vi "Alpha Ver 1.0.vi"() -> ()   [LabVIEW 2015]
uses:
  <instrlib>/Keithley 622x LV 2009/Configure/Source/Typedefs/KE622x -- Current Range.ctl
  <instrlib>/Keithley 622x LV 2009/Configure/Source/Typedefs/KE622x -- Current Ranges.ctl
  <instrlib>/Keithley 622x LV 2009/Typedefs/KE622x -- On Off Control.ctl
  <instrlib>/Keithley 622x LV 2009/Utility/Typedefs/KE622x -- Instrument Type.ctl
  <instrlib>/Keithley 622x LV 2009/Configure/Source/Typedefs/KE622x -- Voltage Limit.ctl
  <instrlib>/Keithley 2000/Public/Configure/Configure DC Volts.vi
  <userlib>/LV-Link3/PolySubVIs/DtCreateAinChan.vi
  <userlib>/LV-Link3/PolySubVIs/DtOLReadSingle.vi
  <instrlib>/Keithley 2000/Keithley 2000.lvlib
  <instrlib>/Keithley 622x LV 2009/Keithley 622x.lvlib
panel:
  out "code":i32
  out "source":string
  out "DAQ A3":dbl format="%#_13g"
  out "DAQ A2":dbl format="%#_13g"
  out "DAQ A1":dbl format="%#_13g"
  out "DAQ cluster":T1
  out "Real stop cur":dbl format="%#_13g"
  out "Real start cur":dbl format="%#_13g"
  in  "Stop cur prefix":u16(ring)
  in  "Start cur prefix":u16(ring)
  out "MULTIPLE GRAPHS":cluster{dbl[], dbl[]}[](graph)
  in  "X-Axis":T2(ring)
  in  "Range":u8(ring)=20 items=["100nV", "200nV", "500nV", "1µV", "2µV", "5µV", "10µV", "20µV", "50µV", "100µV", "200µV", "500µV", "1mV", "2mV", "5mV", "10mV", "20mV", "50mV", "100mV", "200mV", "500mV", "1V"]
  in  "Display Type copy":u16(ring)=3 items=["X %", "Y %", "X Calibrated", "Y Calibrated", "Mag %", "Mag Calibrated", "Phase Degrees", "Ratio", "ADC 1", "ADC 2", "ADC 3", "ADC 4 ", "Noise %", "Noise Calibrated", "Ref Frequency", "", ""]
  out "Units copy":string
  out "Display copy":dbl format="%.3f"
  out "Overload":bool
  out "Display":dbl format="%.3f"
  out "Units":string
  in  "Display Type":u16(ring)=2 items=["X %", "Y %", "X Calibrated", "Y Calibrated", "Mag %", "Mag Calibrated", "Phase Degrees", "Ratio", "ADC 1", "ADC 2", "ADC 3", "ADC 4 ", "Noise %", "Noise Calibrated", "Ref Frequency", "", ""]
  in  "Time Constant":u16(ring) items=["MIN", "1ms", "3ms", "10ms", "30ms", "100ms", "300ms", "1s", "3s", "10s", "30s", "100s", "300s"]
  in  "Slope":u8(ring) items=["6db/octave", "12dB/octave"]
  in  "Dynamic Reserve":u16(ring) items=["High Stability", "Normal", "High Reserve"]
  in  "Auto Sensitivity":bool
  in  "Auto Measure":bool
  out "6221_error_out":errorcluster
  out "2000_error_out":errorcluster
  out "5110_error_out":errorcluster
  out "Input Mode":i32(ring) items=[" Voltage Input (A or A-B) ", "Current Input 10E6 V/A", "Current Input 10E8 V/A"]
  out "5110":refnum<visa-resource-name>
  in  "GPIB Address":i8=11 min=1 max=32 step=1
  out "DAQ A0":dbl format="%#_13g"
  out "2000":dbl format="%#_13g"
  in  "Device":string(combo)
  in  "Number \nof points":i32
  in  "Folder\nprename":string
  out "TIME GRAPH":cluster{dbl[], dbl[]}[](graph)
  out "T0":u32
  out "LIMIT":bool
  out "LIMIT":bool
  out "Error Code":string
  in  "Comments":string
  out "file":refnum<file>
  out "2000":refnum<visa-resource-name>
  out "6221":refnum<visa-resource-name>
  out "Step  (A)":dbl=5e-05 format="%#_3p"
  in  "Stop\ncurrent (A)":dbl=0.002 format="%#_6p"
  in  "Start \ncurrent (A)":dbl=0.001 format="%#_6p"
  in  "Check For SCPI Errors? (T)":bool=TRUE
  out "Interlock Tripped?":bool
  out "Compliance?":bool
  in  "Turn Off Output \nIf Compliance?":bool=TRUE
  in  "Turning ON/OFF\ncurrent output":T3=enum."On"
  in  "Range Selection":T4={"Auto Range?"=TRUE, "Man / Selected\nRange"=enum."2nA"}
  # "FILE CONFIGURATION"
  # "ADMIN PANEL"
  # "KEITHLEY 6221 CONFIGURATION (ADMIN ONLY)"
  # "KEITHLEY DAQ CONFIGURATION (ADMIN ONLY)"
  # "PRINCETON LOCK-IN AMP (ADMIN ONLY)"
  # "I don't know what the hell it is,\njust don't touch it"
  # "SENSITIVITY"
  # "INPUT CONFIGURATION"
  # "READINGS"
  # "START, STOP, STEP, CONFIGURATION"
  # "IF ON"
  # "Output Channels Time - Constant \nSlope & Dynamic Reserve"
  # "Compliance = Limiting output voltage\nThis switch determines if we want to switch \noff the current output if wee exceed compliance"
  # "LOCK-IN READINGS"
  # "RIGHT DISPLAY"
  # "LEFT DISPLAY"
  # "There is a safe switch at \nthe back of the instrument \nThis indicator shows if it is on"
  # "You have hit a damn jackpot \nby exceeding the limited voltage\nCongrats"
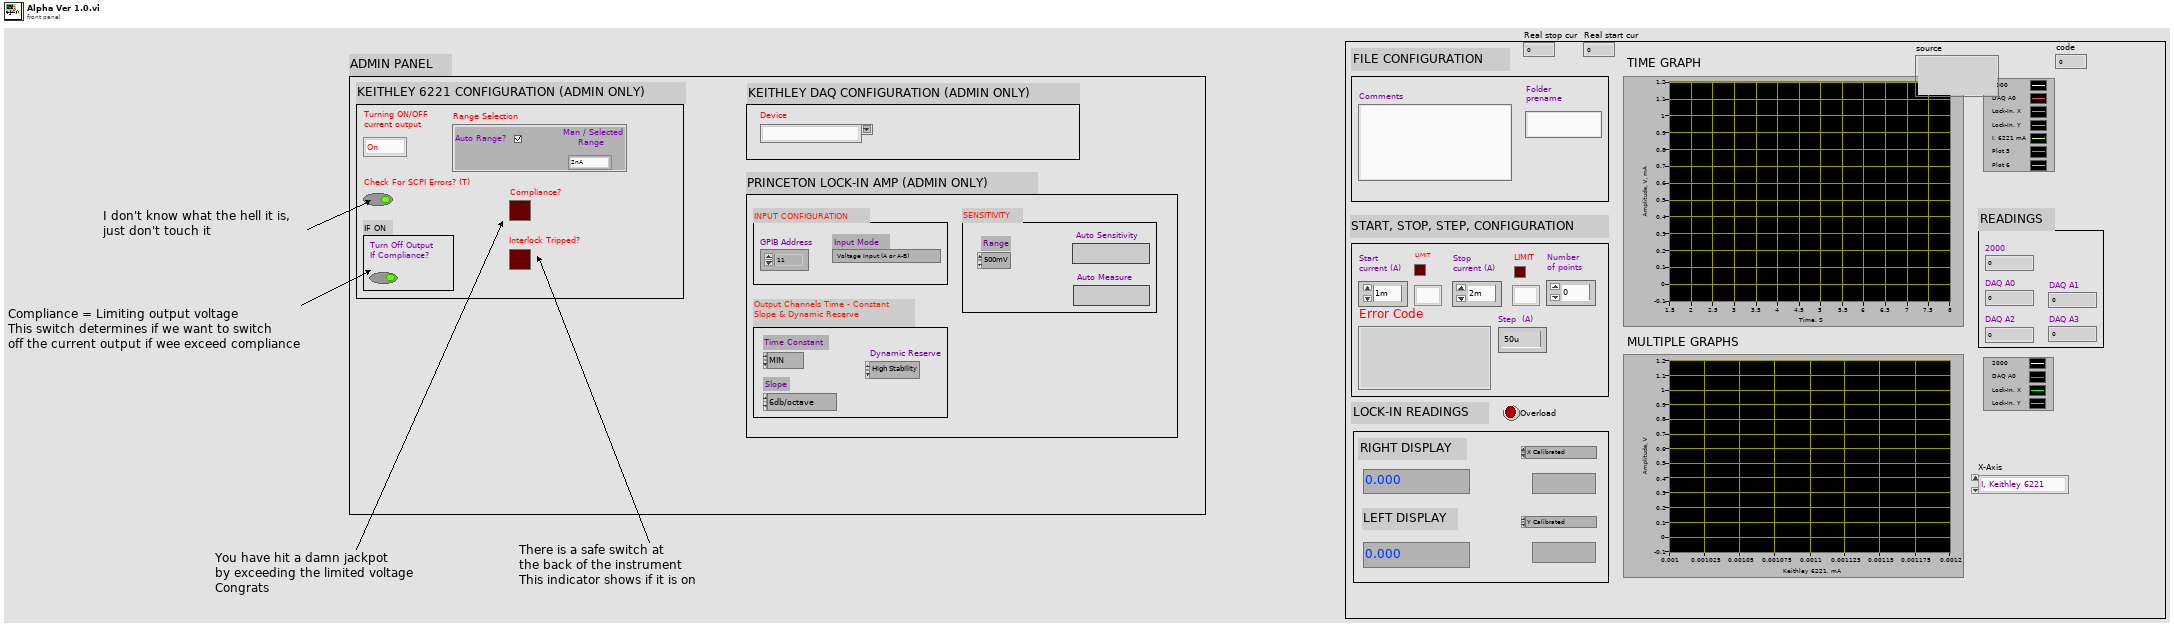
[diagram p1: front panel]
types:
  T1 = cluster{"Task out":i32, "error out":errorcluster, "Task out":i32, "error out":errorcluster, "Task out":i32, "error out":errorcluster, "Task out":i32, "error out":errorcluster}
  T2 = enum16{"I, Keithley 6221", "V, Keithley 2000", "V, Keithley DAQ A0", "V, Keithley DAQ A1", "V, Keithley DAQ A2", "V, Keithley DAQ A3", "V, Lock-In X", "V, Lock-In Y"}
  T3 = typedef "Keithley 622x.lvlib/KE622x -- On Off Control.ctl" = enum16{"Off", "On"}
  T4 = typedef "Keithley 622x.lvlib/KE622x -- Current Range.ctl" = cluster{"Auto Range?":bool, "Man / Selected\nRange":T5}
  T5 = typedef "Keithley 622x.lvlib/KE622x -- Current Ranges.ctl" = enum16{"2nA", "20nA", "200nA", "2uA", "20uA", "200uA", "2mA", "20mA", "100mA"}
  T6 = typedef "Keithley 622x.lvlib/KE622x -- Instrument Type.ctl" = enum16{"KE6220", "KE6221"}
  T7 = typedef "Keithley 622x.lvlib/KE622x -- Voltage Limit.ctl" = dbl
  T8 = cluster{"Data Out":dbl, "Data Out":dbl, "Data Out":dbl, "Data Out":dbl, "Measurement":dbl}
  T9 = cluster{dbl[], dbl[], dbl[], dbl[], dbl[], dbl[], dbl[], dbl[], dbl[]}
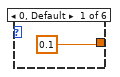
[diagram p2: hidden frame]
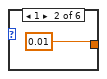
[diagram p3: hidden frame]
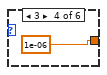
[diagram p4: hidden frame]
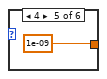
[diagram p5: hidden frame]
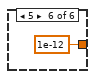
[diagram p6: hidden frame]
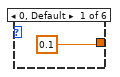
[diagram p7: hidden frame]
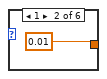
[diagram p8: hidden frame]
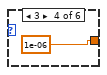
[diagram p9: hidden frame]
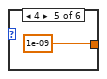
[diagram p10: hidden frame]
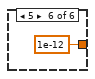
[diagram p11: hidden frame]
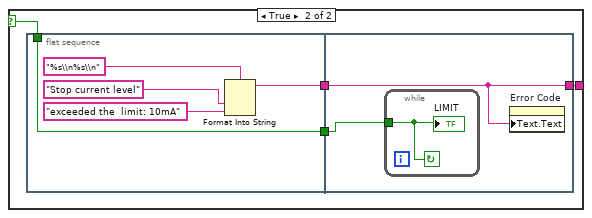
[diagram p12: hidden frame]
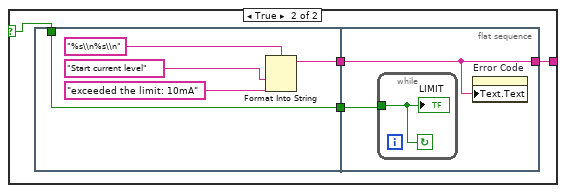
[diagram p13: hidden frame]
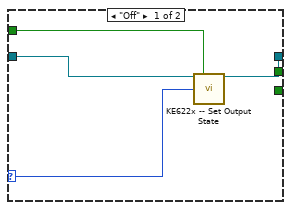
[diagram p14: hidden frame]
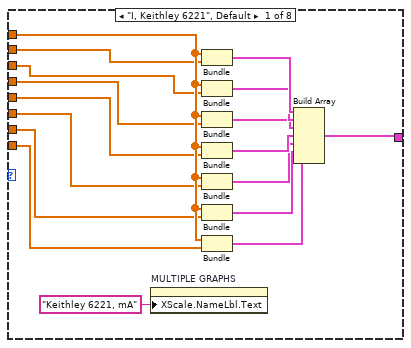
[diagram p15: hidden frame]
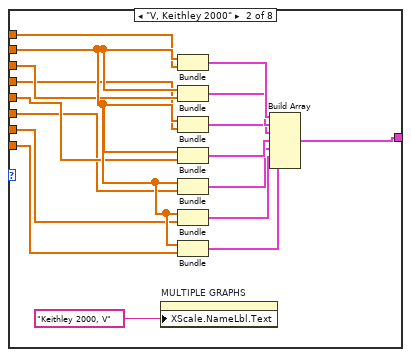
[diagram p16: hidden frame]
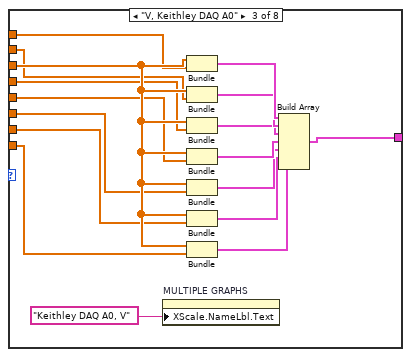
[diagram p17: hidden frame]
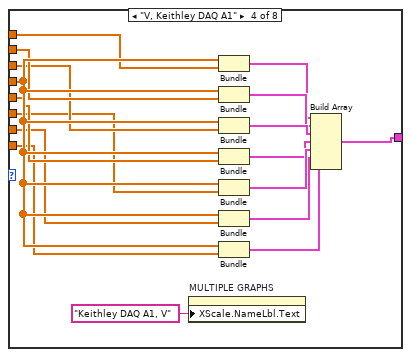
[diagram p18: hidden frame]
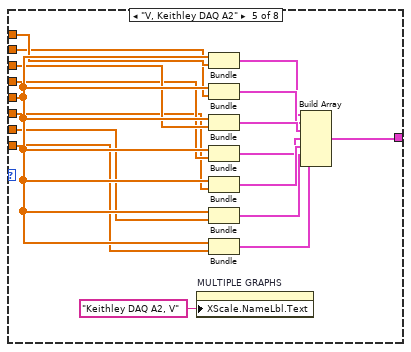
[diagram p19: hidden frame]
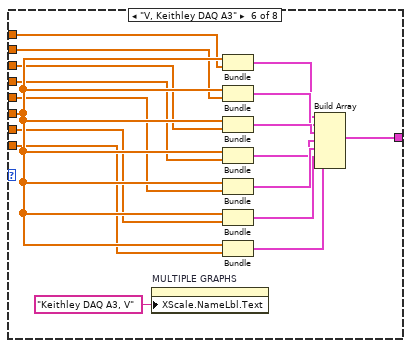
[diagram p20: hidden frame]
diagram:
  n1 = flat-sequence {
    tunnel: [w181] -> w7
    tunnel: [w180] -> w6
    tunnel: [w179] -> w5
    tunnel: [w178] -> w4
    tunnel: [w177] -> w3
    tunnel: [w176] -> w2
    tunnel: [w165] -> w1
    tunnel: w7 -> [w849]
    tunnel: w6 -> [w848]
    tunnel: w5 -> [w847]
    tunnel: w4 -> [w846]
    tunnel: w3 -> [w845]
    tunnel: w2 -> [w844]
    tunnel: w1 -> [w843]
    frame #0 {
      # "File configuration"
      # "Start, Stop, Step"
      # "Time Intit"
      # "Initializing instruments"
      n2 = flat-sequence {
        frame #0 {
          w16 = TRUE  # reset
          w15 = FALSE  # ID query
          # "Initialize Lock-In 5110"
          # "Initialize Keithley 2000"
          # "Initialize Keithley 6221"
          n3 = call <instrlib>:"Initialize.vi"("VISA resource name"=refnum<visa-resource-name> "KEITHLEY_MULTIMETER") -> ("VISA resource name out"=w20:refnum<visa-resource-name>)  [unwired: 17 in, 1 out]
          n4 = call <instrlib>:"Initialize.vi"("VISA resource name"=refnum<visa-resource-name> "KEITHLEY_DC_AC_CURRENT_SOURCE", "Error Queue Option"=enum16{"Clear Error Queue", "Error Query"}."Clear Error Queue", "Instrument Type"=KE622x_--_Instrument_Type."KE6221") -> ("VISA resource name out"=→"6221":refnum<visa-resource-name>, "error out"=→"6221_error_out":errorcluster)  [unwired: 11 in]
          n5 = call "SR51XX Initialize"("VISA session (for class)"=refnum<visa-resource-name> "LOCK_IN_5110_PRINCETON", "Interface"=FALSE, "ID query"=w15, "GPIB Address"="GPIB Address", "reset"=w16) -> ("VISA session"=→"5110":refnum<visa-resource-name>, "error out"=→"5110_error_out":errorcluster)  [unwired: 8 in, 1 out]
          n6 = call-poly <instrlib>:"Configure Measurement.vi"("VISA resource name"=w20) -> ("VISA resource name out"=→"2000":refnum<visa-resource-name>, "error out"=→"2000_error_out":errorcluster)  [unwired: 17 in]
        }
        frame #1 {
          # "Initialize Keithley DAQ \n(getting board name)"
          n7 = call <userlib>:"DtOLGetBoardNames.vi"() -> ("Number of boards"=w25:u32)  [unwired: 9 in, 2 out]
          n8 = Initialize Array("", w25) -> (w27:string[])
          n9 = for {
            N: w25 -> [_]
            shift-right: [w33] -> w30
            shift-left: w27 -> [w34]
            i -> [w32]
            n10 = Add(x=1, y=w32) -> (x+y=w36:i32)
            n11 = call <userlib>:"DtOLGetBoardNames.vi"("Select Board"=w36) -> ("Board Name"=w31:string)  [unwired: 8 in, 2 out]
            n12 = Replace Array Subset(array=w34, new element=w31, index=w32) -> (w33:string[])
          }
          n13 = Index Array(array=w30, index=0) -> (element=w29:string)
          n14 = property on="Device" class="CmbBox"("Strings[]"=w30, "Value"=w29) -> ()  [unwired: 2 in, 2 out]
        }
        frame #2 {
          # "Calculating steps by number\nof points"
          # "Putting in a loop \ninstead of \"STOP\""
          n15 = local read "Real stop cur"() -> (w53:dbl)
          n16 = local read "Real start cur"() -> (w54:dbl)
          n17 = case shown="2" "Start cur prefix" {
            tunnel: [0.1 0.01 0.001 1e-06 1e-09 1e-12] -> w42
            frame 0, Default {
            }
            frame 1 {
            }
            frame 2 {
            }
            frame 3 {
            }
            frame 4 {
            }
            frame 5 {
            }
          }
          n18 = case shown="2" "Stop cur prefix" {
            tunnel: [0.1 0.01 0.001 1e-06 1e-09 1e-12] -> w40
            frame 0, Default {
            }
            frame 1 {
            }
            frame 2 {
            }
            frame 3 {
            }
            frame 4 {
            }
            frame 5 {
            }
          }
          n19 = Subtract(x=w53, y=w54) -> (x-y=w56:dbl)
          n20 = Multiply(x=w42, y="Start \ncurrent (A)") -> (x*y=w38:dbl)
          "Real start cur" <- w38
          n21 = Divide(x=w56, y="Number \nof points") -> (x/y=→"Step  (A)":dbl)
          n22 = Multiply(x=w40, y="Stop\ncurrent (A)") -> (x*y=w37:dbl)
          "Real stop cur" <- w37
          n23 = Greater?(x=w37, y=T7 0.01) -> (0:w48:bool)
          n24 = Greater?(x=w38, y=T7 0.01) -> (0:w47:bool)
          n25 = case shown="False" w48 {
            selector: w48 -> [_ w72]
            tunnel: [w69 w75] -> w50
            frame False {
              n26 = Format Into String(format string="%s\\n", "Start current level is OK" ("false string")) -> (resulting string=w69:string)  [unwired: 2 in, 1 out]
            }
            frame True {
              n27 = flat-sequence {
                tunnel: [w77] -> w74
                tunnel: [w76] -> w73
                tunnel: w72 -> [w76]
                tunnel: [w81] -> w75
                tunnel: w74 -> [w81]
                tunnel: w73 -> [w82]
                frame #0 {
                  n28 = Format Into String(format string="%s\\n%s\\n", "Stop current level" ("String"), "exceeded the  limit: 10mA" ("input 2")) -> (resulting string=w77:string)  [unwired: 2 in, 1 out]
                }
                frame #1 {
                  n29 = while {
                    tunnel: w82 -> [w83]
                    stop <- w83 continue-if-true
                    "LIMIT" <- w83
                  }
                  n30 = property on="Error Code" class="Str"("Text.Text"=w81) -> ()  [unwired: 2 in, 2 out]
                }
              }
            }
          }
          n31 = case shown="False" w47 {
            selector: w47 -> [_ w88]
            tunnel: [w84 w90] -> w49
            frame False {
              n32 = Format Into String(format string="%s\\n", "Start current level is OK" ("false string")) -> (resulting string=w84:string)  [unwired: 2 in, 1 out]
            }
            frame True {
              n33 = flat-sequence {
                tunnel: [w92] -> w89
                tunnel: w88 -> [w91]
                tunnel: [w91] -> w87
                tunnel: [w96] -> w90
                tunnel: w89 -> [w96]
                tunnel: w87 -> [w97]
                frame #0 {
                  n34 = Format Into String(format string="%s\\n%s\\n", "Start current level" ("String"), "exceeded the limit: 10mA" ("input 2")) -> (resulting string=w92:string)  [unwired: 2 in, 1 out]
                }
                frame #1 {
                  n35 = while {
                    tunnel: w97 -> [w98]
                    stop <- w98 continue-if-true
                    "LIMIT" <- w98
                  }
                  n36 = property on="Error Code" class="Str"("Text.Text"=w96) -> ()  [unwired: 2 in, 2 out]
                }
              }
            }
          }
          n37 = Concatenate Strings(w49, w50) -> (→"Error Code":string)
        }
        frame #3 {
          n38 = flat-sequence {
            frame #0 {
              # "Creating folder&file"
              n39 = call "folder_creation.vi"("Name"="Folder\nprename") -> ("String"=w100:string)
              n40 = call "file_creation.vi"("String"=w100) -> ("refnum out"=→"file":refnum<file>)
            }
            frame #1 {
              # "Creating comments"
              n41 = local read "file"() -> (w102:refnum<file>)
              n42 = Format Into String(format string="# %s\\n", initial string=w102, "Comments") -> ()  [unwired: 1 in, 2 out]
            }
            frame #2 {
              # "Writing instr params"
              n43 = local read "5110"() -> (w110:refnum<visa-resource-name>)
              n44 = local read "Real stop cur"() -> (w108:dbl)
              n45 = local read "file"() -> (w105:refnum<file>)
              n46 = local read "Real start cur"() -> (w109:dbl)
              n47 = call "com_inst.vi"("Stop current"=w108, "Start current"=w109, "VISA session (for class)"=w110) -> ("concatenated string"=w106:string)
              n48 = Format Into String(format string="# %s\\n", initial string=w105, w106) -> ()  [unwired: 1 in, 2 out]
            }
            frame #3 {
              # "Adding headlines"
              n49 = local read "file"() -> (w121:refnum<file>)
              n50 = Format Into String(format string="# %-6s  %-12s %-12s %-12s %-12s %-12s  %-12s %-14s %-14s\\n", initial string=w121, "t, ms" ("input 3"), "2000, V" ("input 1"), "DAQ A0" ("input 2"), "DAQ A1" ("input 2"), "DAQ A2" ("input 2"), "DAQ A3" ("input 2"), "5110_X" ("input 3"), "5110_Y " ("input 3"), "6221, mA" ("input 3")) -> ()  [unwired: 1 in, 2 out]
            }
          }
        }
      }
      n51 = Tick Count (ms)() -> (millisecond timer value=→"T0":u32)
    }
    frame #1 {
      # "Configuring Keithley DAQ just before measuments"
      # "Configuring Keithley 6221 just before measuments"
      n52 = flat-sequence {
        tunnel: [w140] -> w122
        tunnel: [w158] -> _
        tunnel: [w160] -> _
        tunnel: w122 -> [w159]
        frame #0 {
          # "Current range \nselection check"
          # "Checking for compliance\nand interlock errors"
          n53 = local read "6221"() -> (w143:refnum<visa-resource-name>)
          n54 = call <instrlib>:"KE622x -- Set Current Range.vi"("Resource In"=w143, "Current Range In"="Range Selection", "Read Back Set Values? (T)"=FALSE) -> ("Resource Out (dupl)"=w148:refnum<visa-resource-name>)  [unwired: 10 in, 2 out]
          n55 = case shown="\"On\"" "Turning ON/OFF\ncurrent output" {
            selector: "Turning ON/OFF\ncurrent output" -> [w152 _]
            tunnel: [_ w156] -> w146
            tunnel: [_ w155] -> w147
            tunnel: "Check For SCPI Errors? (T)" -> [w151 _]
            tunnel: w148 -> [w149 w154]
            tunnel: [w150 w153] -> w140
            frame "Off" {
              n56 = call <instrlib>:"KE622x -- Set Output State.vi"("Resource In"=w149, "Check For SCPI Errors? (T)"=w151, "Output State"=w152) -> ("Resource Out (dupl)"=w150:refnum<visa-resource-name>)  [unwired: 11 in, 1 out]
            }
            frame "On" {
              n57 = call <instrlib>:"KE622x -- Turn Output On And Check For Errors.vi"("Resource In"=w154, "Turn Off Output If Compliance?"="Turn Off Output \nIf Compliance?") -> ("Resource Out (dupl)"=w153:refnum<visa-resource-name>, "Interlock Tripped?"=w156:bool, "Compliance?"=w155:bool)  [unwired: 10 in, 1 out]
            }
          }
          "Interlock Tripped?" <- w146
          "Compliance?" <- w147
        }
        frame #1 {
          # "Setting start current"
          n58 = local read "Real start cur"() -> (w158:dbl)
          n59 = Wait (ms)(milliseconds to wait=u32 100) -> ()  [unwired: 1 out]
          n60 = call <instrlib>:"KE622x -- Set Current Level.vi"("Resource In"=w159, "Current Level (A) In"=w158) -> ("Resource Out (dupl)"=w160:refnum<visa-resource-name>)  [unwired: 12 in, 1 out]
        }
      }
      n61 = flat-sequence {
        frame #0 {
          w134 = 10.0 ("Range Max")
          w133 = -10.0 ("Range Min")
          w135 = 100 items=["SingleEnded"=100, "Differential"=101] ("Channel Type")
          # "Configure the input channel"
          n62 = call-poly <userlib>:"DtOLCreateTask.vi"("Channel Type"=w135, "Range Min"=w133, "Range Max"=w134, "Board Name"="Device", "Channel"="0" ("Channels")) -> ("Task out"=w131:i32, "error out"=w130:errorcluster)  [unwired: 8 in, 1 out]
          n63 = call-poly <userlib>:"DtOLCreateTask.vi"("Channel Type"=w135, "Range Min"=w133, "Range Max"=w134, "Board Name"="Device", "Channel"="1") -> ("Task out"=w129:i32, "error out"=w128:errorcluster)  [unwired: 8 in, 1 out]
          n64 = call-poly <userlib>:"DtOLCreateTask.vi"("Channel Type"=w135, "Range Min"=w133, "Range Max"=w134, "Board Name"="Device", "Channel"="2") -> ("Task out"=w127:i32, "error out"=w126:errorcluster)  [unwired: 8 in, 1 out]
          n65 = call-poly <userlib>:"DtOLCreateTask.vi"("Channel Type"=w135, "Range Min"=w133, "Range Max"=w134, "Board Name"="Device", "Channel"="3") -> ("Task out"=w125:i32, "error out"=w124:errorcluster)  [unwired: 8 in, 1 out]
          n66 = Bundle("Task out"=w131, "error out"=w130, "Task out"=w129, "error out"=w128, "Task out"=w127, "error out"=w126, "Task out"=w125, "error out"=w124) -> (→"DAQ cluster":T1)  [unwired: 1 in]
        }
      }
    }
    frame #2 {
      n67 = local read "5110"() -> (w172:refnum<visa-resource-name>)
      n68 = local read "2000"() -> (w171:refnum<visa-resource-name>)
      n69 = local read "6221"() -> (w170:refnum<visa-resource-name>)
      n70 = local read "5110_error_out"() -> (w169:errorcluster)
      n71 = local read "6221_error_out"() -> (w168:errorcluster)
      n72 = local read "2000_error_out"() -> (w167:errorcluster)
      n73 = local read "DAQ cluster"() -> (w166:T1)
      n74 = while {
        shift-right: [w276] -> _
        shift-left: dbl[] [] -> [w444]
        shift-right: [w277] -> _
        shift-left: i32[] [] -> [w443]
        tunnel: w171 -> [w441]
        tunnel: w170 -> [w440]
        shift-right: [w272] -> _
        shift-left: dbl[] [] -> [w433]
        tunnel: [w432] -> w181
        tunnel: [w431] -> w180
        tunnel: [w429] -> w179
        tunnel: [w426] -> w178
        tunnel: w172 -> [w422]
        tunnel: w169 -> [w421]
        tunnel: w168 -> [w413]
        tunnel: w167 -> [w412]
        tunnel: [w363] -> w177
        tunnel: [w360] -> w176
        shift-right: [w271] -> _
        shift-left: dbl[] [] -> [w359]
        shift-right: [w270] -> _
        shift-left: dbl[] [] -> [w358]
        shift-right: [w278] -> _
        shift-left: dbl[] [] -> [w355]
        tunnel: w166 -> [w312]
        tunnel: [w308] -> w165
        shift-right: [w275] -> _
        shift-left: dbl[] [] -> [w307]
        shift-right: [w274] -> _
        shift-left: dbl[] [] -> [w306]
        shift-right: [w273] -> _
        shift-left: dbl[] [] -> [w305]
        i -> [w414]
        stop <- w434 stop-if-true
        # "V, DAQ A3"
        # "V, DAQ A2"
        # "V, DAQ A1"
        # "Y-V, 5110"
        # "X-V, 5110"
        # "I, 6221"
        # "Config delay"
        # "Control subVI 5110"
        # "Read config 5110"
        # "Measurement config 5110"
        # "Time config 5110"
        # "Configuring Right Display 5110"
        # "Configuring Left Display 5110"
        # "Setting 6221 current"
        # "Delay before measuremens"
        # "Getting the data from DAQ and 2000"
        # "Changing input current"
        # "Time"
        # "V, DAQ A0"
        # "V, 2000"
        n75 = local read "T0"() -> (w442:u32)
        n76 = Quotient & Remainder(x=w414, y=10) -> (floor(x/y)=w419:i32)  [unwired: 1 out]
        n77 = Equal?(x=0, y=w414) -> (x = y?=w416:bool)
        n78 = Subtract(x=w403, y=w442) -> (x-y=w323:u32)
        n79 = Equal?(x=1, y=w419) -> (x = y?=w415:bool)
        n80 = flat-sequence {
          tunnel: w441 -> [w591]
          tunnel: [w591] -> w354
          tunnel: w440 -> [w590]
          tunnel: [w590] -> w352
          tunnel: w422 -> [w588]
          tunnel: [w588] -> w350
          tunnel: [w587] -> w348
          tunnel: w421 -> [w587]
          tunnel: w416 -> [w586]
          tunnel: [w586] -> w346
          tunnel: w415 -> [w585]
          tunnel: [w585] -> w344
          tunnel: w413 -> [w584]
          tunnel: [w584] -> w342
          tunnel: w412 -> [w583]
          tunnel: [w583] -> w340
          tunnel: [w582] -> w403
          tunnel: [w581] -> w313
          tunnel: w312 -> [w581]
          tunnel: w354 -> [w606]
          tunnel: [w606] -> w353
          tunnel: w352 -> [w605]
          tunnel: [w605] -> w351
          tunnel: w350 -> [w604]
          tunnel: [w604] -> w349
          tunnel: w348 -> [w603]
          tunnel: [w603] -> w347
          tunnel: w346 -> [w602]
          tunnel: [w602] -> w345
          tunnel: w344 -> [w601]
          tunnel: [w601] -> w343
          tunnel: w342 -> [w600]
          tunnel: [w600] -> w341
          tunnel: w340 -> [w599]
          tunnel: [w599] -> w339
          tunnel: [w592] -> w314
          tunnel: w313 -> [w592]
          tunnel: w353 -> [w619]
          tunnel: [w619] -> w402
          tunnel: w351 -> [w618]
          tunnel: [w618] -> w401
          tunnel: w349 -> [w617]
          tunnel: w347 -> [w614]
          tunnel: [w613] -> w400
          tunnel: [w612] -> w399
          tunnel: w345 -> [w611]
          tunnel: [w611] -> w398
          tunnel: w343 -> [w610]
          tunnel: w341 -> [w609]
          tunnel: [w609] -> w397
          tunnel: w339 -> [w608]
          tunnel: [w608] -> w396
          tunnel: [w607] -> w315
          tunnel: w314 -> [w607]
          tunnel: w402 -> [w644]
          tunnel: [w644] -> w395
          tunnel: w401 -> [w643]
          tunnel: [w643] -> w394
          tunnel: w400 -> [w640]
          tunnel: [w639] -> w393
          tunnel: w399 -> [w638]
          tunnel: [w637] -> w392
          tunnel: w398 -> [w635]
          tunnel: [w635] -> w391
          tunnel: w397 -> [w642]
          tunnel: [w642] -> w390
          tunnel: w396 -> [w641]
          tunnel: [w641] -> w389
          tunnel: ["Auto Measure"] -> w388
          tunnel: ["Auto Sensitivity"] -> w387
          tunnel: [w630] -> w386
          tunnel: [w627] -> w316
          tunnel: w315 -> [w627]
          tunnel: w395 -> [w663]
          tunnel: [w663] -> w338
          tunnel: w394 -> [w662]
          tunnel: [w662] -> w337
          tunnel: w393 -> [w655]
          tunnel: w392 -> [w653]
          tunnel: [w652] -> w336
          tunnel: w391 -> [w659]
          tunnel: [w659] -> w335
          tunnel: w390 -> [w661]
          tunnel: [w661] -> w334
          tunnel: w389 -> [w660]
          tunnel: [w660] -> w333
          tunnel: w388 -> [w657]
          tunnel: [w657] -> w332
          tunnel: w387 -> [w658]
          tunnel: [w658] -> w331
          tunnel: w386 -> [w648]
          tunnel: [w648] -> w330
          tunnel: [w654] -> w329
          tunnel: ["Time Constant"] -> w328
          tunnel: ["Slope"] -> w327
          tunnel: [w645] -> w317
          tunnel: w316 -> [w645]
          tunnel: [w687] -> w385
          tunnel: [w686] -> w384
          tunnel: [w672] -> w383
          tunnel: [w685] -> w382
          tunnel: [w684] -> w381
          tunnel: [w683] -> w380
          tunnel: [w682] -> w379
          tunnel: [w681] -> w378
          tunnel: [w674] -> w377
          tunnel: [w677] -> w376
          tunnel: [w675] -> w375
          tunnel: [w680] -> w374
          tunnel: [w665] -> w293
          tunnel: w327 -> [w680]
          tunnel: w328 -> [w675]
          tunnel: w329 -> [w678]
          tunnel: w330 -> [w674]
          tunnel: w331 -> [w681]
          tunnel: w332 -> [w682]
          tunnel: w333 -> [w683]
          tunnel: w334 -> [w684]
          tunnel: w335 -> [w685]
          tunnel: w336 -> [w673]
          tunnel: w337 -> [w686]
          tunnel: w338 -> [w687]
          tunnel: [w664] -> w318
          tunnel: w317 -> [w664]
          tunnel: w385 -> [w711]
          tunnel: [w711] -> w373
          tunnel: w384 -> [w710]
          tunnel: [w710] -> w372
          tunnel: w383 -> [w697]
          tunnel: w382 -> [w709]
          tunnel: [w709] -> w371
          tunnel: w381 -> [w708]
          tunnel: [w708] -> w370
          tunnel: w380 -> [w707]
          tunnel: [w707] -> w369
          tunnel: w379 -> [w706]
          tunnel: [w706] -> w368
          tunnel: w378 -> [w705]
          tunnel: [w705] -> w367
          tunnel: w377 -> [w698]
          tunnel: w376 -> [w695]
          tunnel: [w694] -> w366
          tunnel: w375 -> [w699]
          tunnel: w374 -> [w700]
          tunnel: [w696] -> w365
          tunnel: [w693] -> w364
          tunnel: [w689] -> w292
          tunnel: [w688] -> w319
          tunnel: w318 -> [w688]
          tunnel: [w715] -> w438
          tunnel: w414 -> [w723]
          tunnel: [w719] -> w434
          tunnel: [w713] -> w436
          tunnel: [w721] -> w435
          tunnel: [w718] -> w411
          tunnel: [w717] -> w410
          tunnel: [w716] -> w409
          tunnel: [w714] -> w408
          tunnel: [w713] -> w294
          tunnel: w364 -> [_]
          tunnel: w365 -> [w716]
          tunnel: w366 -> [w714]
          tunnel: w367 -> [_]
          tunnel: w368 -> [_]
          tunnel: w369 -> [w718]
          tunnel: w370 -> [w717]
          tunnel: w371 -> [_]
          tunnel: w372 -> [w721]
          tunnel: w373 -> [w715]
          tunnel: [w712] -> w320
          tunnel: w319 -> [w712]
          tunnel: w438 -> [w735]
          tunnel: [w735] -> w437
          tunnel: w436 -> [w734]
          tunnel: w435 -> [w733]
          tunnel: [w732] -> w430
          tunnel: [w731] -> w427
          tunnel: w411 -> [w729]
          tunnel: w410 -> [w730]
          tunnel: w409 -> [w727]
          tunnel: w408 -> [w728]
          tunnel: [w729] -> w407
          tunnel: [w728] -> w404
          tunnel: [w727] -> w361
          tunnel: [w726] -> w321
          tunnel: w320 -> [w726]
          tunnel: w437 -> [w743]
          tunnel: [w743] -> w439
          tunnel: w430 -> [w741]
          tunnel: [w741] -> w428
          tunnel: w427 -> [w740]
          tunnel: [w740] -> w425
          tunnel: w407 -> [w739]
          tunnel: [w739] -> w406
          tunnel: [w738] -> w405
          tunnel: w404 -> [w738]
          tunnel: [w737] -> w362
          tunnel: w361 -> [w737]
          tunnel: [w736] -> w322
          tunnel: w321 -> [w736]
          tunnel: w439 -> [w778]
          tunnel: w428 -> [w774]
          tunnel: w425 -> [w773]
          tunnel: w406 -> [w770]
          tunnel: w405 -> [w769]
          tunnel: w362 -> [w768]
          tunnel: w322 -> [w767]
          tunnel: [w771] -> w235
          tunnel: [w772] -> w234
          tunnel: [w776] -> w233
          tunnel: [w775] -> w232
          tunnel: [w774] -> w231
          tunnel: [w773] -> w230
          tunnel: [w772] -> w229
          tunnel: [w771] -> w228
          tunnel: [w769] -> w227
          tunnel: [w768] -> w226
          tunnel: [w746] -> w225
          tunnel: [w745] -> w224
          tunnel: [w744] -> w223
          tunnel: [w747] -> w222
          tunnel: [w746] -> w221
          tunnel: [w745] -> w220
          tunnel: [w744] -> w219
          tunnel: w235 -> [w795]
          tunnel: w234 -> [w794]
          tunnel: w233 -> [w793]
          tunnel: w232 -> [w792]
          tunnel: w231 -> [w791]
          tunnel: w230 -> [w790]
          tunnel: w229 -> [w789]
          tunnel: w228 -> [w788]
          tunnel: w227 -> [w787]
          tunnel: w226 -> [w786]
          tunnel: w225 -> [w785]
          tunnel: w224 -> [w784]
          tunnel: w223 -> [w783]
          tunnel: w222 -> [w782]
          tunnel: w221 -> [w781]
          tunnel: w220 -> [w780]
          tunnel: w219 -> [w779]
          tunnel: [w795] -> w218
          tunnel: [w794] -> w217
          tunnel: [w793] -> w216
          tunnel: [w792] -> w215
          tunnel: [w791] -> w214
          tunnel: [w790] -> w213
          tunnel: [w789] -> w212
          tunnel: [w788] -> w211
          tunnel: [w787] -> w210
          tunnel: [w786] -> w209
          tunnel: [w785] -> w208
          tunnel: [w784] -> w207
          tunnel: [w783] -> w206
          tunnel: [w782] -> w205
          tunnel: [w781] -> w204
          tunnel: [w780] -> w203
          tunnel: [w779] -> w202
          tunnel: w218 -> [w812]
          tunnel: w217 -> [w811]
          tunnel: w216 -> [w810]
          tunnel: w215 -> [w809]
          tunnel: w214 -> [w808]
          tunnel: w213 -> [w807]
          tunnel: w212 -> [w806]
          tunnel: w211 -> [w805]
          tunnel: w210 -> [w804]
          tunnel: w209 -> [w803]
          tunnel: w208 -> [w802]
          tunnel: w207 -> [w801]
          tunnel: w206 -> [w800]
          tunnel: w205 -> [w799]
          tunnel: w204 -> [w798]
          tunnel: w203 -> [w797]
          tunnel: w202 -> [w796]
          tunnel: [w812] -> w201
          tunnel: [w811] -> w200
          tunnel: [w810] -> w199
          tunnel: [w809] -> w198
          tunnel: [w808] -> w197
          tunnel: [w807] -> w196
          tunnel: [w806] -> w195
          tunnel: [w805] -> w194
          tunnel: [w804] -> w193
          tunnel: [w803] -> w192
          tunnel: [w802] -> w191
          tunnel: [w801] -> w190
          tunnel: [w800] -> w189
          tunnel: [w799] -> w188
          tunnel: [w798] -> w187
          tunnel: [w797] -> w186
          tunnel: [w796] -> w185
          tunnel: [w813] -> w301
          tunnel: [w814] -> w302
          tunnel: [w815] -> w303
          tunnel: [w816] -> w308
          tunnel: [w817] -> w309
          tunnel: [w818] -> w310
          tunnel: [w819] -> w311
          tunnel: [w820] -> w360
          tunnel: [w821] -> w363
          tunnel: [w822] -> w423
          tunnel: [w823] -> w424
          tunnel: [w824] -> w426
          tunnel: [w825] -> w429
          tunnel: [w826] -> w431
          tunnel: [w827] -> w432
          tunnel: [w828] -> w304
          tunnel: [w829] -> w300
          tunnel: w201 -> [w829]
          tunnel: w200 -> [w828]
          tunnel: w199 -> [w827]
          tunnel: w198 -> [w826]
          tunnel: w197 -> [w825]
          tunnel: w196 -> [w824]
          tunnel: w195 -> [w823]
          tunnel: w194 -> [w822]
          tunnel: w193 -> [w821]
          tunnel: w192 -> [w820]
          tunnel: w191 -> [w819]
          tunnel: w190 -> [w818]
          tunnel: w189 -> [w817]
          tunnel: w188 -> [w816]
          tunnel: w187 -> [w815]
          tunnel: w186 -> [w814]
          tunnel: w185 -> [w813]
          frame #0 {
            n81 = Wait Until Next ms Multiple(millisecond multiple=u32 500) -> (millisecond timer value=w582:u32)
          }
          frame #1 {
            n82 = control-ref of="Range"() -> (w598:refnum<vi>)
            n83 = control-ref of="Auto Sensitivity"() -> (w597:refnum<vi>)
            n84 = control-ref of="Auto Measure"() -> (w596:refnum<vi>)
            n85 = control-ref of="Time Constant"() -> (w593:refnum<vi>)
            n86 = control-ref of="Slope"() -> (w594:refnum<vi>)
            n87 = control-ref of="Dynamic Reserve"() -> (w595:refnum<vi>)
            n88 = call "cont_ver_1.0.vi"("Dynamic Reserve"=w595, "Slope"=w594, "Time Constant"=w593, "Auto Measure"=w596, "Auto Sensitivity"=w597, "Range"=w598) -> ()
          }
          frame #2 {
            n89 = case shown="False" w610 {
              tunnel: w617 -> [w621 w626]
              tunnel: [w620 w624] -> w616
              tunnel: [w621 w623] -> w615
              tunnel: w614 -> [w620 w622]
              frame False {
              }
              frame True {
                n90 = call "SR51XX Read Preamp Input Mode"("VISA session (for class)"=w626, "error in (no error)"=w622) -> ("VISA session"=w623:refnum<visa-resource-name>, "Input Mode"=w625:i32, "error out"=w624:errorcluster)  [unwired: 15 in]
                n91 = local write "Input Mode"(w625) -> ()
              }
            }
            n92 = call "SR51XX Configure Signal Channel Input"("VISA session (for class)"=w615, "error in (no error)"=w616, "Update"=w611) -> ("VISA session"=w613:refnum<visa-resource-name>, "error out"=w612:errorcluster)  [unwired: 15 in]
          }
          frame #3 {
            n93 = local read "Input Mode"() -> (w636:i32)
            n94 = call "SR51XX Configure Sensitivity"("VISA session (for class)"=w640, "Input Mode"=w636, "Range"="Range", "error in (no error)"=w638, "Auto Sensitivity"="Auto Sensitivity", "Auto Measure"="Auto Measure", "Update"=w635) -> ("Range Annotations Out[]"=w628:string[], "VISA session"=w639:refnum<visa-resource-name>, "Auto Sensitivity out"=w632:bool, "Auto Measure out"=w631:bool, "Range Out"=w630:u8, "error out"=w637:errorcluster)  [unwired: 7 in]
            n95 = property on="Range" class="Ring (strict)"("Strings []"=w628) -> ()  [unwired: 2 in, 2 out]
            n96 = local write "Auto Sensitivity"(w632) -> ()
            n97 = local write "Auto Measure"(w631) -> ()
            n98 = local write "Range"(w630) -> ()
          }
          frame #4 {
            n99 = Or(x=w658, y=w657) -> (x .or. y?=w656:bool)
            n100 = call "SR51XX Configure Output Channels - Slope, TC and Dyn Reserve"("VISA session (for class)"=w655, "Time Constant"="Time Constant", "Slope"="Slope", "Check TC"=w656, "Dynamic Reserve"="Dynamic Reserve", "error in (no error)"=w653, "Range"=w648, "Update"=w659) -> ("VISA session"=w654:refnum<visa-resource-name>, "Slope Out"=w649:u8, "Time Constant Out"=w650:u16, "error out"=w652:errorcluster)  [unwired: 8 in]
            n101 = local write "Slope"(w649) -> ()
            n102 = local write "Time Constant"(w650) -> ()
          }
          frame #5 {
            n103 = local read "Input Mode"() -> (w679:i32)
            n104 = call "SR5110 Read Output"("VISA session (for class)"=w678, "Input Mode"=w679, "Time Constant"=w675, "Display Type"="Display Type", "Range"=w674, "error in (no error)"=w673, "Slope"=w680) -> ("Units"=w667:string, "Display Precision"=w671:i32, "Display"=w666:dbl, "VISA session"=w677:refnum<visa-resource-name>, "Available Display Types Out"=w670:string[], "Overload"=→"Overload":bool, "error out"=w672:errorcluster)  [unwired: 4 in, 2 out]
            "Units" <- w667
            "Display" <- w666
            n105 = property on="Display Type" class="Ring (strict)"("Strings []"=w670) -> ()  [unwired: 2 in, 2 out]
            n106 = property on="Display" class="DigNum (strict)"("Precision"=w671) -> ()  [unwired: 2 in, 2 out]
            n107 = call "pref_to_num.vi"("string"=w667) -> ("Numeric"=w668:dbl)
            n108 = Multiply(x=w668, y=w666) -> (x*y=w665:dbl)
          }
          frame #6 {
            n109 = local read "Input Mode"() -> (w704:i32)
            n110 = call "SR5110 Read Output"("VISA session (for class)"=w695, "Input Mode"=w704, "Time Constant"=w699, "Display Type"="Display Type copy", "Range"=w698, "error in (no error)"=w697, "Slope"=w700) -> ("Units"=w692:string, "Display Precision"=w701:i32, "Display"=w691:dbl, "VISA session"=w694:refnum<visa-resource-name>, "Reference Unlock"=w693:bool, "Available Display Types Out"=w702:string[], "error out"=w696:errorcluster)  [unwired: 4 in, 2 out]
            "Display copy" <- w691
            "Units copy" <- w692
            n111 = property on="Display Type copy" class="Ring (strict)"("Strings []"=w702) -> ()  [unwired: 2 in, 2 out]
            n112 = property on="Display copy" class="DigNum (strict)"("Precision"=w701) -> ()  [unwired: 2 in, 2 out]
            n113 = call "pref_to_num.vi"("string"=w692) -> ("Numeric"=w690:dbl)
            n114 = Multiply(x=w690, y=w691) -> (x*y=w689:dbl)
          }
          frame #7 {
            n115 = local read "Step  (A)"() -> (w724:dbl)
            n116 = local read "Real start cur"() -> (w725:dbl)
            n117 = Multiply(x=w724, y=w723) -> (x*y=w722:dbl)
            n118 = Add(x=w725, y=w722) -> (x+y=w713:dbl)
            n119 = local read "Real stop cur"() -> (w720:dbl)
            n120 = Greater Or Equal?(x=w713, y=w720) -> (x >= y?=w719:bool)
          }
          frame #8 {
            n121 = call <instrlib>:"KE622x -- Set Current Level.vi"("Resource In"=w733, "Current Level (A) In"=w734, "error in (no error)"=w730) -> ("Resource Out (dupl)"=w731:refnum<visa-resource-name>, "error out"=w732:errorcluster)  [unwired: 11 in]
          }
          frame #9 {
            n122 = Wait Until Next ms Multiple(millisecond multiple=u32 50) -> ()  [unwired: 1 out]
          }
          frame #10 {
            n123 = Unbundle(w767) -> ("Task out"=w766:i32, "error out"=w765:errorcluster, "Task out"=w763:i32, "error out"=w762:errorcluster, "Task out"=w760:i32, "error out"=w759:errorcluster, "Task out"=w758:i32, "error out"=w757:errorcluster)
            n124 = call <instrlib>:"Data Read Single.vi"("VISA resource name"=w778, "error in (no error)"=w770) -> ("VISA resource name out"=w775:refnum<visa-resource-name>, "Measurement"=w771:dbl, "error out"=w776:errorcluster)  [unwired: 13 in, 2 out]
            n125 = call-poly <userlib>:"DtOLRead.vi"("error in (no error)"=w765, "Timeout"=1.0, "Task in"=w766) -> ("error out"=w754:errorcluster, "Data Out"=w772:dbl, "Task out"=w755:i32)  [unwired: 6 in]
            n126 = call-poly <userlib>:"DtOLRead.vi"("error in (no error)"=w757, "Timeout"=1.0, "Task in"=w758) -> ("error out"=w748:errorcluster, "Data Out"=w744:dbl, "Task out"=w749:i32)  [unwired: 6 in]
            n127 = call-poly <userlib>:"DtOLRead.vi"("error in (no error)"=w762, "Timeout"=1.0, "Task in"=w763) -> ("error out"=w752:errorcluster, "Data Out"=w746:dbl, "Task out"=w753:i32)  [unwired: 6 in]
            n128 = call-poly <userlib>:"DtOLRead.vi"("error in (no error)"=w759, "Timeout"=1.0, "Task in"=w760) -> ("error out"=w750:errorcluster, "Data Out"=w745:dbl, "Task out"=w751:i32)  [unwired: 6 in]
            n129 = Bundle("Task out"=w755, "error out"=w754, "Task out"=w753, "error out"=w752, "Task out"=w751, "error out"=w750, "Task out"=w749, "error out"=w748) -> (w747:T1)  [unwired: 1 in]
          }
          frame #11 {
          }
          frame #12 {
          }
          frame #13 {
          }
        }
        n130 = Divide(x=w323, y=u32 1000) -> (x/y=w324:dbl)
        n131 = Build Array (concatenate)(w443, w324) -> (w286:dbl[])
        n132 = local read "file"() -> (w326:refnum<file>)
        n133 = Bundle(w294, w293, w292) -> (w291:cluster{dbl, dbl, dbl})  [unwired: 1 in]
        n134 = Unbundle(w291) -> (w290:dbl, w289:dbl, w288:dbl)
        n135 = Build Array (concatenate)(w355, w290) -> (w287:dbl[])
        n136 = Build Array (concatenate)(w359, w289) -> (w280:dbl[])
        n137 = Build Array (concatenate)(w358, w288) -> (w279:dbl[])
        n138 = Bundle("Data Out"=w304, "Data Out"=w303, "Data Out"=w302, "Data Out"=w301, "Measurement"=w300) -> (w241:T8)  [unwired: 1 in]
        n139 = Unbundle(w241) -> ("Data Out"=w298:dbl, "Data Out"=w297:dbl, "Data Out"=w296:dbl, "Data Out"=w295:dbl, "Measurement"=w299:dbl)
        n140 = Unbundle(w241) -> ("Data Out"=w239:dbl, "Data Out"=w238:dbl, "Data Out"=w237:dbl, "Data Out"=w236:dbl, "Measurement"=w240:dbl)
        n141 = Build Array (concatenate)(w444, w299) -> (w285:dbl[])
        n142 = Build Array (concatenate)(w307, w298) -> (w284:dbl[])
        n143 = Build Array (concatenate)(w306, w297) -> (w283:dbl[])
        n144 = Build Array (concatenate)(w305, w296) -> (w282:dbl[])
        n145 = Build Array (concatenate)(w433, w295) -> (w281:dbl[])
        n146 = Format Into String(format string="%08d  %8.2e %12g %14.5e %12.4e %12.4e\\n", initial string=w326, w323, w240, w239, w238, w237, w236) -> ()  [unwired: 1 in, 2 out]
        n147 = Bundle(w287, w286, w285, w284, w283, w282, w281, w280, w279) -> (w251:T9)  [unwired: 1 in]
        n148 = Unbundle(w251) -> (w261:dbl[], w269:dbl[], w268:dbl[], w267:dbl[], w266:dbl[], w265:dbl[], w264:dbl[], w263:dbl[], w262:dbl[])
        n149 = Bundle(w269, w268) -> (w260:cluster{dbl[], dbl[]})  [unwired: 1 in]
        n150 = Bundle(w269, w267) -> (w259:cluster{dbl[], dbl[]})  [unwired: 1 in]
        n151 = Bundle(w269, w266) -> (w258:cluster{dbl[], dbl[]})  [unwired: 1 in]
        n152 = Bundle(w269, w265) -> (w257:cluster{dbl[], dbl[]})  [unwired: 1 in]
        n153 = Bundle(w269, w264) -> (w256:cluster{dbl[], dbl[]})  [unwired: 1 in]
        n154 = Bundle(w269, w263) -> (w255:cluster{dbl[], dbl[]})  [unwired: 1 in]
        n155 = Bundle(w269, w262) -> (w254:cluster{dbl[], dbl[]})  [unwired: 1 in]
        n156 = Bundle(w269, w261) -> (w253:cluster{dbl[], dbl[]})  [unwired: 1 in]
        n157 = Build Array(w260, w259, w258, w257, w256, w255, w254, w253) -> (→"TIME GRAPH":cluster{dbl[], dbl[]}[])
        n158 = Unbundle(w251) -> (w250:dbl[], w249:dbl[], w248:dbl[], w247:dbl[], w246:dbl[], w245:dbl[], w244:dbl[], w243:dbl[])  [unwired: 1 out]
        n159 = case shown="\"V, Lock-In Y\"" "X-Axis" {
          tunnel: [w445 w470 w487 w496 w521 w538 w555 w572] -> w242
          tunnel: w250 -> [w460 w468 w485 w503 w519 w536 w553 w570]
          tunnel: w249 -> [w459 w469 w484 w502 w518 w535 w552 w569]
          tunnel: w248 -> [w458 w467 w486 w501 w517 w534 w551 w568]
          tunnel: w247 -> [w457 w466 w483 w504 w516 w533 w550 w567]
          tunnel: w246 -> [w456 w465 w482 w500 w520 w532 w549 w566]
          tunnel: w245 -> [w455 w464 w481 w499 w515 w537 w548 w565]
          tunnel: w244 -> [w454 w463 w480 w498 w514 w531 w554 w564]
          tunnel: w243 -> [w453 w462 w479 w497 w513 w530 w547 w571]
          frame "I, Keithley 6221", Default {
            n160 = property on="MULTIPLE GRAPHS" class="XYGraph (strict)"("XScale.NameLbl.Text"="Keithley 6221, mA" ("X Scale.Name Label.Text")) -> ()  [unwired: 2 in, 2 out]
            n161 = Bundle(w460, w459) -> (w452:cluster{dbl[], dbl[]})  [unwired: 1 in]
            n162 = Bundle(w460, w458) -> (w451:cluster{dbl[], dbl[]})  [unwired: 1 in]
            n163 = Bundle(w460, w457) -> (w450:cluster{dbl[], dbl[]})  [unwired: 1 in]
            n164 = Bundle(w460, w456) -> (w449:cluster{dbl[], dbl[]})  [unwired: 1 in]
            n165 = Bundle(w460, w455) -> (w448:cluster{dbl[], dbl[]})  [unwired: 1 in]
            n166 = Bundle(w460, w454) -> (w447:cluster{dbl[], dbl[]})  [unwired: 1 in]
            n167 = Bundle(w460, w453) -> (w446:cluster{dbl[], dbl[]})  [unwired: 1 in]
            n168 = Build Array(w452, w451, w450, w449, w448, w447, w446) -> (w445:cluster{dbl[], dbl[]}[])
          }
          frame "V, Keithley 2000" {
            n169 = property on="MULTIPLE GRAPHS" class="XYGraph (strict)"("XScale.NameLbl.Text"="Keithley 2000, V" ("X Scale.Name Label.Text")) -> ()  [unwired: 2 in, 2 out]
            n170 = Bundle(w469, w468) -> (w477:cluster{dbl[], dbl[]})  [unwired: 1 in]
            n171 = Bundle(w469, w467) -> (w476:cluster{dbl[], dbl[]})  [unwired: 1 in]
            n172 = Bundle(w469, w466) -> (w475:cluster{dbl[], dbl[]})  [unwired: 1 in]
            n173 = Bundle(w469, w465) -> (w474:cluster{dbl[], dbl[]})  [unwired: 1 in]
            n174 = Bundle(w469, w464) -> (w473:cluster{dbl[], dbl[]})  [unwired: 1 in]
            n175 = Bundle(w469, w463) -> (w472:cluster{dbl[], dbl[]})  [unwired: 1 in]
            n176 = Bundle(w469, w462) -> (w471:cluster{dbl[], dbl[]})  [unwired: 1 in]
            n177 = Build Array(w477, w476, w475, w474, w473, w472, w471) -> (w470:cluster{dbl[], dbl[]}[])
          }
          frame "V, Keithley DAQ A0" {
            n178 = property on="MULTIPLE GRAPHS" class="XYGraph (strict)"("XScale.NameLbl.Text"="Keithley DAQ A0, V" ("X Scale.Name Label.Text")) -> ()  [unwired: 2 in, 2 out]
            n179 = Bundle(w486, w485) -> (w494:cluster{dbl[], dbl[]})  [unwired: 1 in]
            n180 = Bundle(w486, w484) -> (w493:cluster{dbl[], dbl[]})  [unwired: 1 in]
            n181 = Bundle(w486, w483) -> (w492:cluster{dbl[], dbl[]})  [unwired: 1 in]
            n182 = Bundle(w486, w482) -> (w491:cluster{dbl[], dbl[]})  [unwired: 1 in]
            n183 = Bundle(w486, w481) -> (w490:cluster{dbl[], dbl[]})  [unwired: 1 in]
            n184 = Bundle(w486, w480) -> (w489:cluster{dbl[], dbl[]})  [unwired: 1 in]
            n185 = Bundle(w486, w479) -> (w488:cluster{dbl[], dbl[]})  [unwired: 1 in]
            n186 = Build Array(w494, w493, w492, w491, w490, w489, w488) -> (w487:cluster{dbl[], dbl[]}[])
          }
          frame "V, Keithley DAQ A1" {
            n187 = property on="MULTIPLE GRAPHS" class="XYGraph (strict)"("XScale.NameLbl.Text"="Keithley DAQ A1, V" ("X Scale.Name Label.Text")) -> ()  [unwired: 2 in, 2 out]
            n188 = Bundle(w504, w503) -> (w506:cluster{dbl[], dbl[]})  [unwired: 1 in]
            n189 = Bundle(w504, w502) -> (w507:cluster{dbl[], dbl[]})  [unwired: 1 in]
            n190 = Bundle(w504, w501) -> (w508:cluster{dbl[], dbl[]})  [unwired: 1 in]
            n191 = Bundle(w504, w500) -> (w509:cluster{dbl[], dbl[]})  [unwired: 1 in]
            n192 = Bundle(w504, w499) -> (w510:cluster{dbl[], dbl[]})  [unwired: 1 in]
            n193 = Bundle(w504, w498) -> (w511:cluster{dbl[], dbl[]})  [unwired: 1 in]
            n194 = Bundle(w504, w497) -> (w512:cluster{dbl[], dbl[]})  [unwired: 1 in]
            n195 = Build Array(w506, w507, w508, w509, w510, w511, w512) -> (w496:cluster{dbl[], dbl[]}[])
          }
          frame "V, Keithley DAQ A2" {
            n196 = property on="MULTIPLE GRAPHS" class="XYGraph (strict)"("XScale.NameLbl.Text"="Keithley DAQ A2, V" ("X Scale.Name Label.Text")) -> ()  [unwired: 2 in, 2 out]
            n197 = Bundle(w520, w519) -> (w522:cluster{dbl[], dbl[]})  [unwired: 1 in]
            n198 = Bundle(w520, w518) -> (w523:cluster{dbl[], dbl[]})  [unwired: 1 in]
            n199 = Bundle(w520, w517) -> (w524:cluster{dbl[], dbl[]})  [unwired: 1 in]
            n200 = Bundle(w520, w516) -> (w525:cluster{dbl[], dbl[]})  [unwired: 1 in]
            n201 = Bundle(w520, w515) -> (w526:cluster{dbl[], dbl[]})  [unwired: 1 in]
            n202 = Bundle(w520, w514) -> (w527:cluster{dbl[], dbl[]})  [unwired: 1 in]
            n203 = Bundle(w520, w513) -> (w528:cluster{dbl[], dbl[]})  [unwired: 1 in]
            n204 = Build Array(w522, w523, w524, w525, w526, w527, w528) -> (w521:cluster{dbl[], dbl[]}[])
          }
          frame "V, Keithley DAQ A3" {
            n205 = property on="MULTIPLE GRAPHS" class="XYGraph (strict)"("XScale.NameLbl.Text"="Keithley DAQ A3, V" ("X Scale.Name Label.Text")) -> ()  [unwired: 2 in, 2 out]
            n206 = Bundle(w537, w536) -> (w539:cluster{dbl[], dbl[]})  [unwired: 1 in]
            n207 = Bundle(w537, w535) -> (w540:cluster{dbl[], dbl[]})  [unwired: 1 in]
            n208 = Bundle(w537, w534) -> (w541:cluster{dbl[], dbl[]})  [unwired: 1 in]
            n209 = Bundle(w537, w533) -> (w542:cluster{dbl[], dbl[]})  [unwired: 1 in]
            n210 = Bundle(w537, w532) -> (w543:cluster{dbl[], dbl[]})  [unwired: 1 in]
            n211 = Bundle(w537, w531) -> (w544:cluster{dbl[], dbl[]})  [unwired: 1 in]
            n212 = Bundle(w537, w530) -> (w545:cluster{dbl[], dbl[]})  [unwired: 1 in]
            n213 = Build Array(w539, w540, w541, w542, w543, w544, w545) -> (w538:cluster{dbl[], dbl[]}[])
          }
          frame "V, Lock-In X" {
            n214 = property on="MULTIPLE GRAPHS" class="XYGraph (strict)"("XScale.NameLbl.Text"="Lock-In X, V" ("X Scale.Name Label.Text")) -> ()  [unwired: 2 in, 2 out]
            n215 = Bundle(w554, w553) -> (w556:cluster{dbl[], dbl[]})  [unwired: 1 in]
            n216 = Bundle(w554, w552) -> (w557:cluster{dbl[], dbl[]})  [unwired: 1 in]
            n217 = Bundle(w554, w551) -> (w558:cluster{dbl[], dbl[]})  [unwired: 1 in]
            n218 = Bundle(w554, w550) -> (w559:cluster{dbl[], dbl[]})  [unwired: 1 in]
            n219 = Bundle(w554, w549) -> (w560:cluster{dbl[], dbl[]})  [unwired: 1 in]
            n220 = Bundle(w554, w548) -> (w561:cluster{dbl[], dbl[]})  [unwired: 1 in]
            n221 = Bundle(w554, w547) -> (w562:cluster{dbl[], dbl[]})  [unwired: 1 in]
            n222 = Build Array(w556, w557, w558, w559, w560, w561, w562) -> (w555:cluster{dbl[], dbl[]}[])
          }
          frame "V, Lock-In Y" {
            n223 = property on="MULTIPLE GRAPHS" class="XYGraph (strict)"("XScale.NameLbl.Text"="Lock-In Y, V" ("X Scale.Name Label.Text")) -> ()  [unwired: 2 in, 2 out]
            n224 = Bundle(w571, w570) -> (w579:cluster{dbl[], dbl[]})  [unwired: 1 in]
            n225 = Bundle(w571, w569) -> (w578:cluster{dbl[], dbl[]})  [unwired: 1 in]
            n226 = Bundle(w571, w568) -> (w577:cluster{dbl[], dbl[]})  [unwired: 1 in]
            n227 = Bundle(w571, w567) -> (w576:cluster{dbl[], dbl[]})  [unwired: 1 in]
            n228 = Bundle(w571, w566) -> (w575:cluster{dbl[], dbl[]})  [unwired: 1 in]
            n229 = Bundle(w571, w565) -> (w574:cluster{dbl[], dbl[]})  [unwired: 1 in]
            n230 = Bundle(w571, w564) -> (w573:cluster{dbl[], dbl[]})  [unwired: 1 in]
            n231 = Build Array(w579, w578, w577, w576, w575, w574, w573) -> (w572:cluster{dbl[], dbl[]}[])
          }
        }
        "MULTIPLE GRAPHS" <- w242
        n232 = Unbundle(w251) -> (w278:dbl[], w277:dbl[], w276:dbl[], w275:dbl[], w274:dbl[], w273:dbl[], w272:dbl[], w271:dbl[], w270:dbl[])
        "2000" <- w423
        "DAQ A0" <- w424
        "DAQ A1" <- w311
        "DAQ A2" <- w310
        "DAQ A3" <- w309
      }
    }
    frame #3 {
      # "Closing instrumental \nconnections"
      n233 = Unbundle(w843) -> ("Task out"=w840:i32, "error out"=w839:errorcluster, "Task out"=w838:i32, "error out"=w837:errorcluster, "Task out"=w836:i32, "error out"=w835:errorcluster, "Task out"=w834:i32, "error out"=w833:errorcluster)
      n234 = call <instrlib>:"Close.vi"("VISA resource name"=w848, "error in (no error)"=w849) -> ()  [unwired: 17 in, 1 out]
      n235 = call "SR51XX Close"("error in (no error)"=w844, "VISA session"=w845) -> ()  [unwired: 1 out]
      n236 = call <instrlib>:"Close.vi"("VISA resource name"=w846, "error in (no error)"=w847) -> ()  [unwired: 13 in, 1 out]
      n237 = call <userlib>:"DtOLCloseTask.vi"("Error in"=w839, "Task in"=w840) -> ("Error Out"=w850:errorcluster)  [unwired: 9 in]
      n238 = call <userlib>:"DtOLCloseTask.vi"("Error in"=w837, "Task in"=w838) -> ("Error Out"=w832:errorcluster)  [unwired: 9 in]
      n239 = call <userlib>:"DtOLCloseTask.vi"("Error in"=w835, "Task in"=w836) -> ("Error Out"=w842:errorcluster)  [unwired: 9 in]
      n240 = call <userlib>:"DtOLCloseTask.vi"("Error in"=w833, "Task in"=w834) -> ("Error Out"=w841:errorcluster)  [unwired: 9 in]
      n241 = call <vilib>:"Simple Error Handler.vi"("error in (no error)"=w850) -> ()  [unwired: 4 in, 5 out]
      n242 = call <vilib>:"Simple Error Handler.vi"("error in (no error)"=w842) -> ()  [unwired: 4 in, 5 out]
      n243 = call <vilib>:"Simple Error Handler.vi"("error in (no error)"=w841) -> ()  [unwired: 4 in, 5 out]
      n244 = Unbundle(w832) -> ("code"=→"code":i32, "source"=→"source":string)  [unwired: 1 out]
      n245 = call <vilib>:"Simple Error Handler.vi"("error in (no error)"=w832) -> ()  [unwired: 4 in, 5 out]
    }
  }
